vi "Exercises_5-2.vi"() -> ()   [LabVIEW 2014]
panel:
  out "Numeric":dbl
  out "Small Cluster":cluster{"Boolean 1":bool, "Slide Value":dbl}
  out "Boolean 2":bool
  in  "stop":bool
  out "Modified Cluster":T1 {"Slide" scale=0.0..10.0}
  in  "Cluster":T1 {"Slide" scale=0.0..10.0}
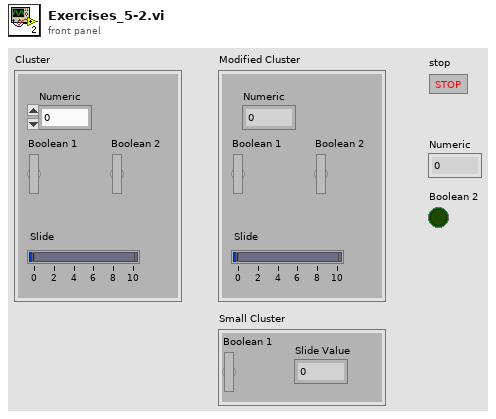
[diagram p1: front panel]
types:
  T1 = cluster{"Numeric":dbl, "Boolean 1":bool, "Boolean 2":bool, "Slide":dbl}
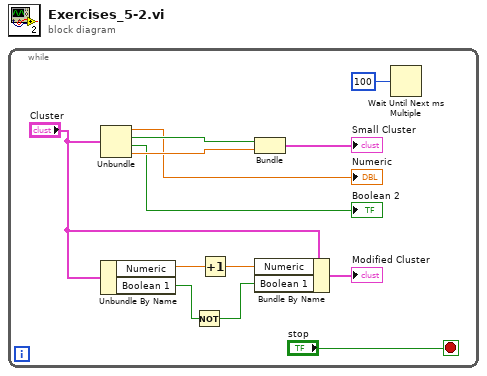
[diagram p0: block diagram]
diagram:
  n1 = while {
    stop <- "stop" stop-if-true
    n2 = Unbundle("Cluster") -> ("Numeric"=→"Numeric":dbl, "Boolean 1"=w7:bool, "Boolean 2"=→"Boolean 2":bool, "Slide"=w6:dbl)
    n3 = Unbundle By Name("Cluster") -> ("Numeric"=w8:dbl, "Boolean 1"=w9:bool)
    n4 = Not(x=w9) -> (.not. x?=w10:bool)
    n5 = Increment(x=w8) -> (x+1=w11:dbl)
    n6 = Bundle("Boolean 1"=w7, "Slide"=w6) -> (→"Small Cluster":cluster{"Boolean 1":bool, "Slide":dbl})  [unwired: 1 in]
    n7 = Bundle By Name(cluster="Cluster", "Numeric"=w11, "Boolean 1"=w10) -> (→"Modified Cluster":T1)
    n8 = Wait Until Next ms Multiple(millisecond multiple=u32 100) -> ()  [unwired: 1 out]
  }
